vi "ParseDeltaTiming.vi"(6 "TermChar (80h)":u8=128 format="%x", 8 "error in (no error)":errorcluster, 11 "Byte Stream File in":refnum<file>) -> (0 "error out":errorcluster, 2 "Delta Time":u32, 3 "Byte Stream File out":refnum<file>)   [LabVIEW 2016]
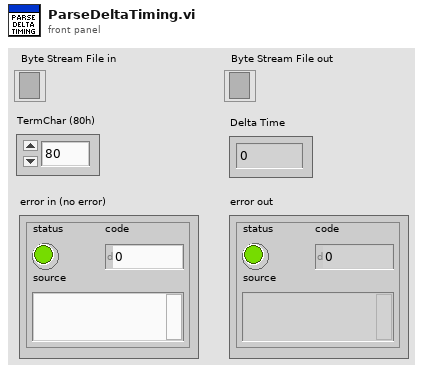
[diagram p1: front panel]
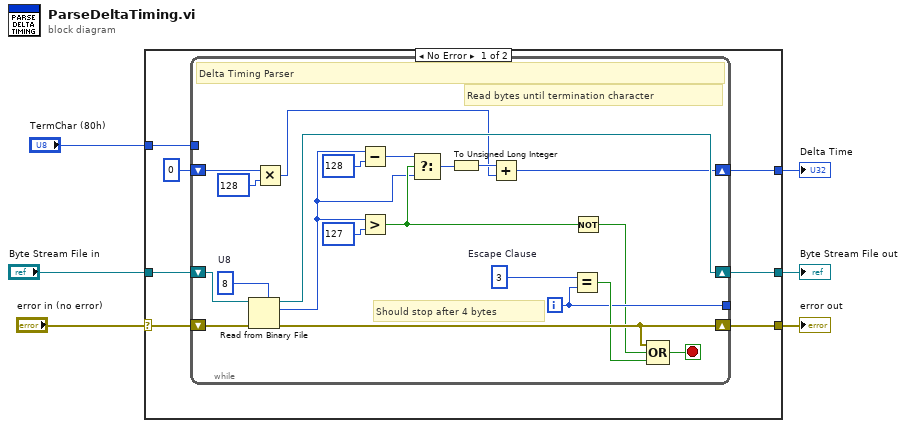
[diagram p0: block diagram]
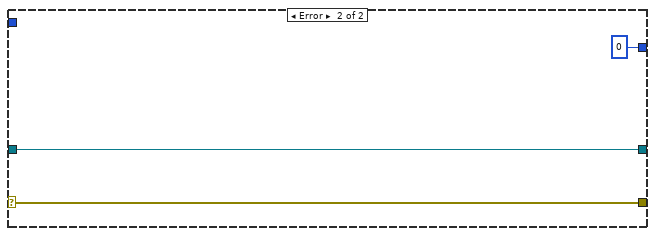
[diagram p2: hidden frame]
diagram:
  n1 = case shown="No Error" "error in (no error)" {
    selector: "error in (no error)" -> [w9 w35]
    tunnel: [w7 u32 0] -> w6
    tunnel: [w13 w36] -> w5
    tunnel: [w12 w35] -> w4
    tunnel: "Byte Stream File in" -> [w10 w36]
    tunnel: "TermChar (80h)" -> [w8 _]
    frame No Error {
      n2 = while {
        shift-right: [w32] -> w13
        shift-left: w10 -> [w34]
        shift-right: [w30] -> w12
        shift-left: w9 -> [w33]
        shift-right: [w17] -> w7
        shift-left: u32 0 -> [w15]
        tunnel: w8 -> [_]
        tunnel: [w26] -> _
        i -> [w26]
        stop <- w31 stop-if-true
        w27 = u8 8  # U8
        w29 = 3  # Escape Clause
        # "Should stop after 4 bytes"
        # "Read bytes until termination character"
        # "Delta Timing Parser"
        n3 = Read from Binary File(5:w27, 8:w33, 11:w34) -> (0:w30:errorcluster, 2:w21:u8, 3:w32:refnum<file>)  [unwired: 3 in, 1 out]
        n4 = Multiply(x=w15, y=u32 128) -> (x*y=w16:u32)
        n5 = Subtract(x=w21, y=u8 128) -> (x-y=w22:u8)
        n6 = Greater?(x=w21, y=u8 127) -> (0:w23:bool)
        n7 = Select(t=w22, s=w23, f=w21) -> (s? t:f=w19:u8)
        n8 = To Unsigned Long Integer(number=w19) -> (unsigned 32bit integer=w18:u32)
        n9 = Add(x=w18, y=w16) -> (x+y=w17:u32)
        n10 = Equal?(x=w29, y=w26) -> (x = y?=w28:bool)
        n11 = Not(x=w23) -> (.not. x?=w20:bool)
        n12 = Compound Arithmetic op=OR(w30, w20, w28) -> (w31:bool)
      }
    }
    frame Error {
    }
  }
  "Delta Time" <- w6
  "Byte Stream File out" <- w5
  "error out" <- w4
